vi "gran linear region.vi"(8 "min points":u8, 9 "sensitivity":dbl=1.0 min=1.0 max=3.0 step=0.01 format="%.2f", 10 "Va":dbl[](array[numeric]) format="%.7f", 11 "F1":dbl[](array[numeric]) format="%.7f") -> (2 "first i":u8, 3 "length":u8)   [LabVIEW 2012]
uses:
  <vilib>/Analysis/NI_AALPro.lvlib
panel:
  in  "minimum F1":dbl=5e-05 format="%.5f"
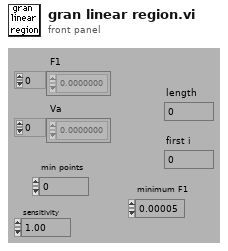
[diagram p1: front panel]
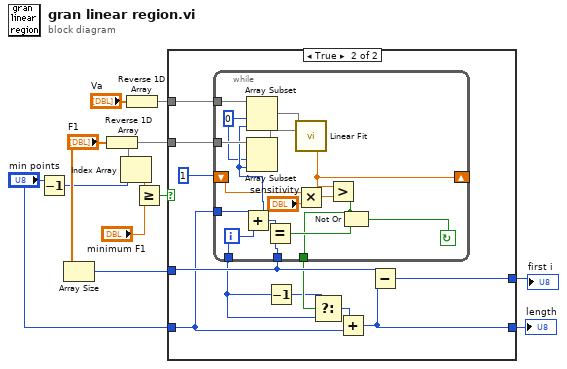
[diagram p0: block diagram]
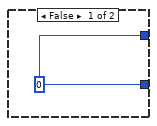
[diagram p2: hidden frame]
diagram:
  n1 = Decrement(x="min points") -> (x-1=w1:u8)
  n2 = Array Size(array="F1") -> (size(s)=w3:i32)
  n3 = Reverse 1D Array(array="F1") -> (reversed array=w10:dbl[])
  n4 = Index Array(array=w10, index=w1) -> (element=w9:dbl)
  n5 = Reverse 1D Array(array="Va") -> (reversed array=w4:dbl[])
  n6 = Greater Or Equal?(x=w9, y="minimum F1") -> (x >= y?=w7:bool)
  n7 = case shown="True" w7 {
    tunnel: [w13 w21] -> w6
    tunnel: [w13 w22] -> w5
    tunnel: w4 -> [_ w24]
    tunnel: w10 -> [_ w23]
    tunnel: w3 -> [_ w20]
    tunnel: "min points" -> [_ w14]
    frame False {
      w13 = 0
    }
    frame True {
      n8 = while {
        tunnel: [w26] -> w17
        tunnel: w20 -> [w30]
        shift-left: 1 -> [w32]
        shift-right: [w31] -> _
        tunnel: w14 -> [w33]
        tunnel: w23 -> [w39]
        tunnel: w24 -> [w40]
        tunnel: [w38] -> w15
        i -> [w38]
        stop <- w29 continue-if-true
        w36 = 0
        n9 = Add(x=w33, y=w38) -> (x+y=w37:i32)
        n10 = Array Subset(array=w40, index=w36, length=w37) -> (w35:dbl[])
        n11 = Array Subset(array=w39, index=w36, length=w37) -> (w34:dbl[])
        n12 = Equal?(x=w37, y=w30) -> (x = y?=w27:bool)
        n13 = call <vilib>:"Linear Fit.vi"("Y"=w35, "X"=w34) -> ("residue"=w31:dbl)  [unwired: 9 in, 4 out]
        n14 = Multiply(x=w32, y="sensitivity") -> (x*y=w28:dbl)
        n15 = Greater?(x=w31, y=w28) -> (0:w26:bool)
        n16 = Not Or(1:w27, 2:w26) -> (0:w29:bool)
      }
      n17 = Decrement(x=w15) -> (x-1=w16:i32)
      n18 = Select(t=w16, s=w17, f=w15) -> (s? t:f=w18:i32)
      n19 = Add(x=w18, y=w14) -> (x+y=w21:i32)
      n20 = Subtract(x=w20, y=w21) -> (x-y=w22:i32)
    }
  }
  "first i" <- w5
  "length" <- w6
